vi "logThermal.vi"(6 "Temp Readings":T1 {"Ambient Temp (°F)" format="%.2f °F"; "Ambient Temp (°C)" format="%.2f °C"; "Object Temp (°F)" format="%.2f °F"; "Object Temp (°C)" format="%.2f °C"}, 8 "Online":bool, 9 "Index":i32) -> ()   [LabVIEW 2014]
uses:
  Type Defs/tempReadings.ctl
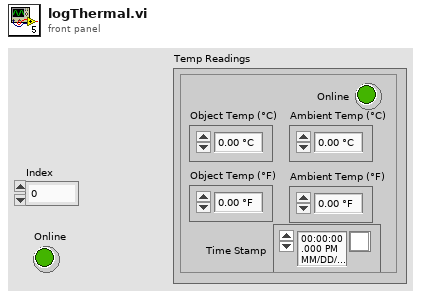
[diagram p1: front panel]
types:
  T1 = typedef "tempReadings.ctl" = cluster{"Object Temp (°C)":dbl, "Object Temp (°F)":dbl, "Ambient Temp (°C)":dbl, "Ambient Temp (°F)":dbl, "Online":bool, "Time Stamp":timestamp}
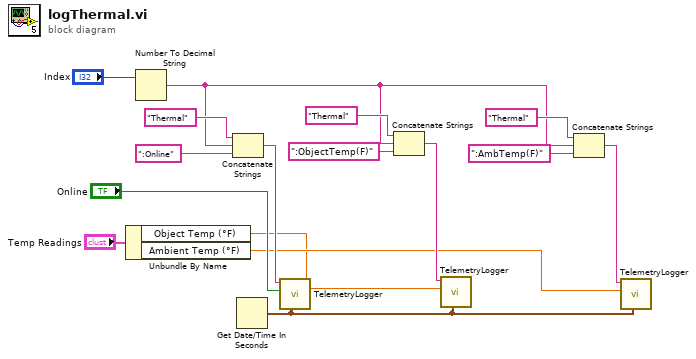
[diagram p0: block diagram]
diagram:
  n1 = Unbundle By Name("Temp Readings") -> ("Object Temp (°F)"=w1:dbl, "Ambient Temp (°F)"=w2:dbl)
  n2 = Number To Decimal String(number="Index") -> (decimal integer string=w5:string)  [unwired: 1 in]
  n3 = Concatenate Strings("Thermal", w5, ":Online") -> (w12:string)
  n4 = Get Date/Time In Seconds() -> (seconds since 1Jan1904=w4:timestamp)
  n5 = call "TelemetryLogger.vi"("Time Stamp"=w4, "Data"="Online", "Sensor:Reading"=w12) -> ()  [unwired: 9 in]
  n6 = Concatenate Strings("Thermal", w5, ":ObjectTemp(F)") -> (w11:string)
  n7 = call "TelemetryLogger.vi"("Time Stamp"=w4, "Data"=w1, "Sensor:Reading"=w11) -> ()  [unwired: 9 in]
  n8 = Concatenate Strings("Thermal", w5, ":AmbTemp(F)") -> (w6:string)
  n9 = call "TelemetryLogger.vi"("Time Stamp"=w4, "Data"=w2, "Sensor:Reading"=w6) -> ()  [unwired: 9 in]
